vi "Simple Timed Logger.vi"() -> ()   [LabVIEW 2017]
panel:
  out "Logging Time":dbl
  in  "Program Stop":bool
  in  "Stop Log Button":bool
  in  "Log button":bool
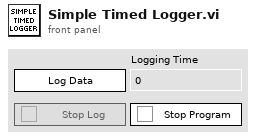
[diagram p1: front panel]
types:
  T1 = cluster{"Start Time":timestamp, "State":enum16{"Waiting", "Logging", "Start Logging", "End Logging"}, "Stop":bool}
  T2 = enum8{"Enabled", "Disabled", "Disabled and Grayed Out"}
  T3 = enum16{"Waiting", "Logging", "Start Logging", "End Logging"}
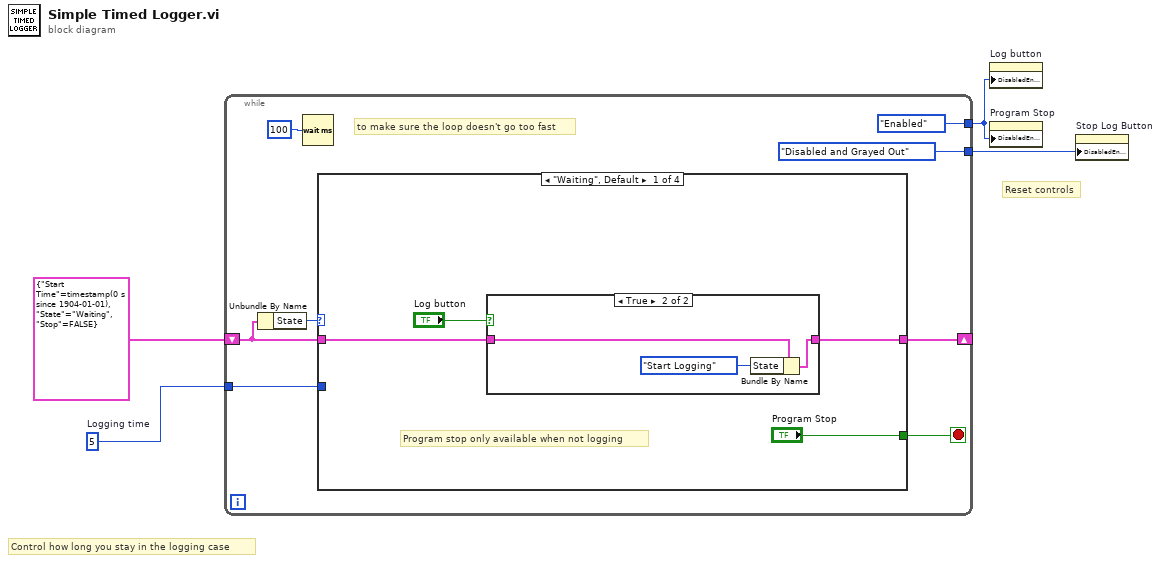
[diagram p0: block diagram]
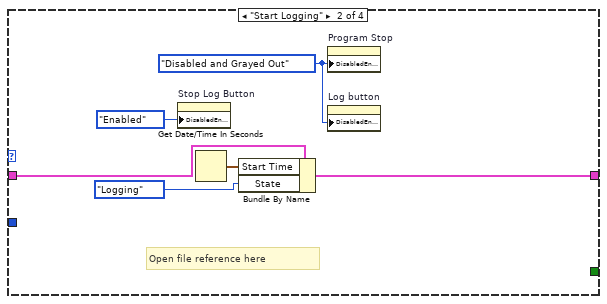
[diagram p3: hidden frame]
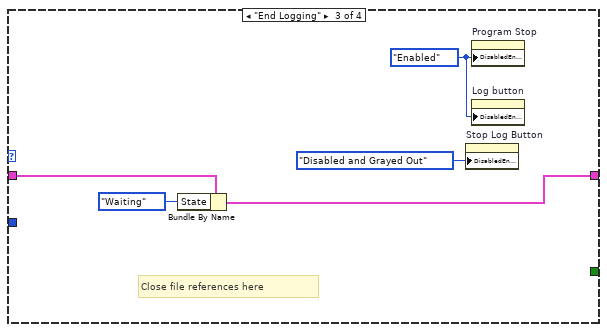
[diagram p4: hidden frame]
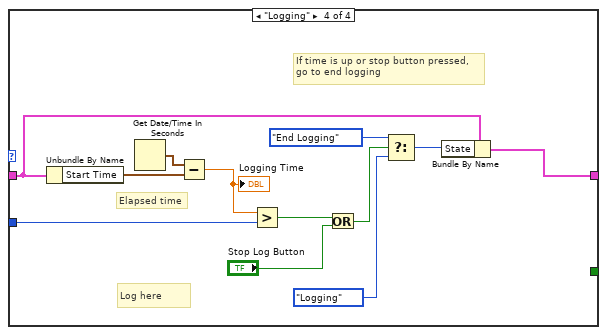
[diagram p5: hidden frame]
diagram:
  w3 = 5  # Logging time
  # "Reset controls"
  # "Control how long you stay in the logging case"
  n1 = while {
    shift-right: [w9] -> _
    shift-left: T1 {"Start Time"=timestamp(0 s since 1904-01-01), "State"=enum."Waiting", "Stop"=FALSE} -> [w11]
    tunnel: w3 -> [w10]
    tunnel: [T2."Disabled and Grayed Out" ("Disabled")] -> w2
    tunnel: [T2."Enabled" ("Disabled")] -> w1
    stop <- w5 stop-if-true
    # "to make sure the loop doesn't go too fast"
    n2 = Unbundle By Name(w11) -> ("State"=w12:T3)
    n3 = Wait (ms)(milliseconds to wait=u32 100) -> ()  [unwired: 1 out]
    n4 = case shown="\"Waiting\", Default" w12 {
      tunnel: [w15 w25 w30 w38] -> w9
      tunnel: w11 -> [w14 w26 w31 w43]
      tunnel: w10 -> [_ _ _ w39]
      tunnel: ["Program Stop" _ _ _] -> w5
      frame "Waiting", Default {
        # "Program stop only available when not logging"
        n5 = case shown="True" "Log button" {
          tunnel: [w17 w19] -> w15
          tunnel: w14 -> [w17 w20]
          frame False {
          }
          frame True {
            n6 = Bundle By Name(cluster=w20, "State"=T3."Start Logging") -> (w19:T1)
          }
        }
      }
      frame "Start Logging" {
        w21 = T2."Disabled and Grayed Out" ("Disabled")
        # "Open file reference here"
        n7 = property on="Stop Log Button" class="Bool"("DisabledEnum"=T2."Enabled" ("Disabled")) -> ()  [unwired: 2 in, 2 out]
        n8 = Get Date/Time In Seconds() -> (seconds since 1Jan1904=w24:timestamp)
        n9 = Bundle By Name(cluster=w26, "Start Time"=w24, "State"=T3."Logging") -> (w25:T1)
        n10 = property on="Program Stop" class="Bool"("DisabledEnum"=w21) -> ()  [unwired: 2 in, 2 out]
        n11 = property on="Log button" class="Bool"("DisabledEnum"=w21) -> ()  [unwired: 2 in, 2 out]
      }
      frame "End Logging" {
        w27 = T2."Enabled" ("Disabled")
        # "Close file references here"
        n12 = Bundle By Name(cluster=w31, "State"=T3."Waiting") -> (w30:T1)
        n13 = property on="Stop Log Button" class="Bool"("DisabledEnum"=T2."Disabled and Grayed Out" ("Disabled")) -> ()  [unwired: 2 in, 2 out]
        n14 = property on="Program Stop" class="Bool"("DisabledEnum"=w27) -> ()  [unwired: 2 in, 2 out]
        n15 = property on="Log button" class="Bool"("DisabledEnum"=w27) -> ()  [unwired: 2 in, 2 out]
      }
      frame "Logging" {
        # "Elapsed time"
        # "If time is up or stop button pressed,\ngo to end logging"
        # "Log here"
        n16 = Unbundle By Name(w43) -> ("Start Time"=w41:timestamp)
        n17 = Get Date/Time In Seconds() -> (seconds since 1Jan1904=w42:timestamp)
        n18 = Subtract(x=w42, y=w41) -> (x-y=w40:dbl)
        "Logging Time" <- w40
        n19 = Greater?(x=w40, y=w39) -> (0:w37:bool)
        n20 = Or(x=w37, y="Stop Log Button") -> (x .or. y?=w33:bool)
        n21 = Select(t=T3."End Logging" ("State"), s=w33, f=T3."Logging" ("State")) -> (s? t:f=w34:T3)
        n22 = Bundle By Name(cluster=w43, "State"=w34) -> (w38:T1)
      }
    }
  }
  n23 = property on="Log button" class="Bool"("DisabledEnum"=w1) -> ()  [unwired: 2 in, 2 out]
  n24 = property on="Program Stop" class="Bool"("DisabledEnum"=w1) -> ()  [unwired: 2 in, 2 out]
  n25 = property on="Stop Log Button" class="Bool"("DisabledEnum"=w2) -> ()  [unwired: 2 in, 2 out]
